vi "Tree Has Node.vi"(8 "error in (no error)":errorcluster, 9 "Path":string, 11 "Tree DVR in":refnum<data-value>) -> (0 "error out":errorcluster, 2 "Is readonly?":bool, 3 "Tree DVR out":refnum<data-value>)   [LabVIEW 2012, in "MDSplus.lvlib"]
uses:
  <vilib>/MDSplus/Library/MDSplus.lvlib
  <vilib>/MDSplus/Classes/Tree_Class/Tree.lvclass
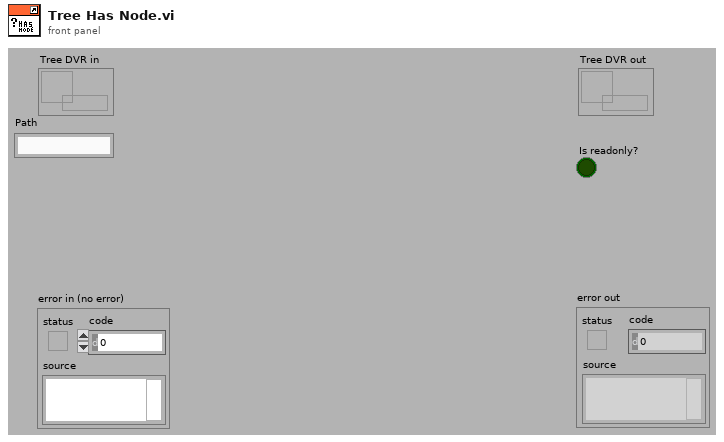
[diagram p1: front panel]
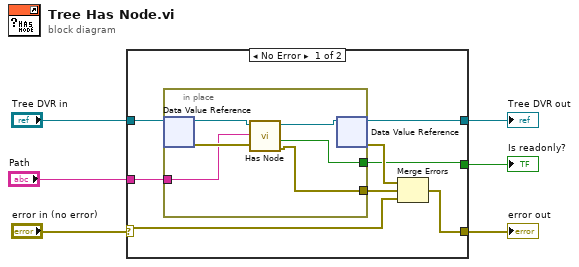
[diagram p0: block diagram]
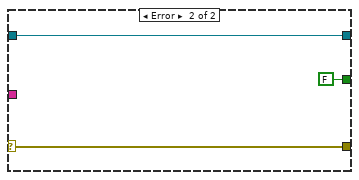
[diagram p2: hidden frame]
diagram:
  n1 = case shown="No Error" "error in (no error)" {
    selector: "error in (no error)" -> [w7 w23]
    tunnel: "Tree DVR in" -> [w14 w22]
    tunnel: [w12 w23] -> w6
    tunnel: [w11 w22] -> w3
    tunnel: [w10 FALSE ("Is modified?")] -> w2
    tunnel: "Path" -> [w9 _]
    frame No Error {
      n2 = in-place {
        in-place-border: [w17] -> w10
        in-place-border: w9 -> [w16]
        in-place-border: [w15] -> w8
        n3 = in-place-dvr #1(w14) -> (w20:refnum<class "Tree.lvclass">, w18:errorcluster)
        n4 = call-dynamic "Has Node.vi"("error in (no error)"=w18, "Path"=w16, "Tree in"=w20) -> ("error out"=w15:errorcluster, "Has Node"=w17:bool, "Tree out"=w19:refnum<class "Tree.lvclass">)  [unwired: 6 in]
        n5 = in-place-dvr #1(w19) -> (w11:refnum<data-value>, w13:errorcluster)
      }
      n6 = Merge Errors(w13, w8, w7) -> (w12:errorcluster)
    }
    frame Error {
    }
  }
  "error out" <- w6
  "Tree DVR out" <- w3
  "Is readonly?" <- w2
